vi "Generate write queue item.vi"(8 "error in (no error)":errorcluster, 10 "Request ID":u64, 11 "Register JSON in":refnum<class "Register JSON.lvclass">) -> (0 "error out":errorcluster, 2 "Write queue item":T1, 3 "Register JSON out":refnum<class "Register JSON.lvclass">)   [LabVIEW 2020, in "wamplv.lvlib" / "Register JSON.lvclass"]
uses:
  Register JSON.lvclass
  Register JSON.lvclass/Register JSON.ctl
  TypeDefs/WAMP Message Codes.ctl
  wamplv.lvlib
  Utils/Utils.lvclass
  91faa4a0-8572-4326-99ac-79b83bae1e0d.vi
  TypeDefs/Transport type.ctl
  WAMP Client/Private/TypeDef/Write queue item.ctl
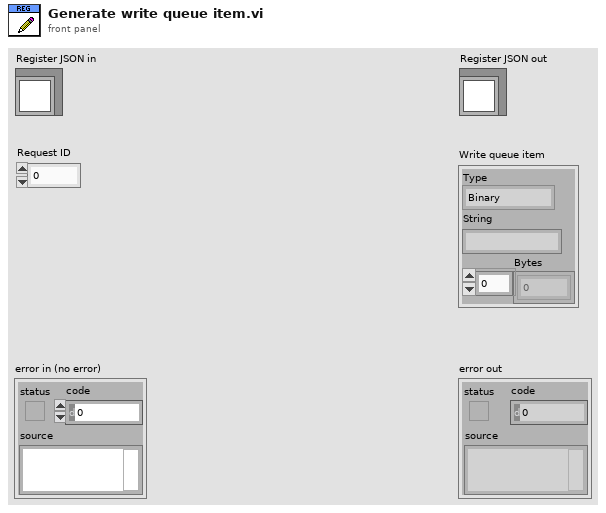
[diagram p1: front panel]
types:
  T1 = typedef "wamplv.lvlib/Write queue item.ctl" = cluster{"Type":T2, "String":string, "Bytes":u8[]}
  T2 = typedef "wamplv.lvlib/Transport type.ctl" = enum16{"Binary", "Text"}
  T3 = typedef "wamplv.lvlib/WAMP Message Codes.ctl" = enum8{"HELLO", "WELCOME", "CHALLENGE", "AUTHENTICATE", "ABORT", "GOODBYE", "ERROR", "PUBLISH", "PUBLISHED", "SUBSCRIBE", "SUBSCRIBED", "UNSUBSCRIBE", "UNSUBSCRIBED", "EVENT", "CALL", "RESULT", "REGISTER", "REGISTERED", "UNREGISTER", "UNREGISTERED", "INVOCATION", "YIELD"}
  T4 = typedef "wamplv.lvlib/REGISTER Request Data.ctl" = cluster{"Procedure URI":string, "Options":string, "REGISTER result notifier":refnum<notifier>}
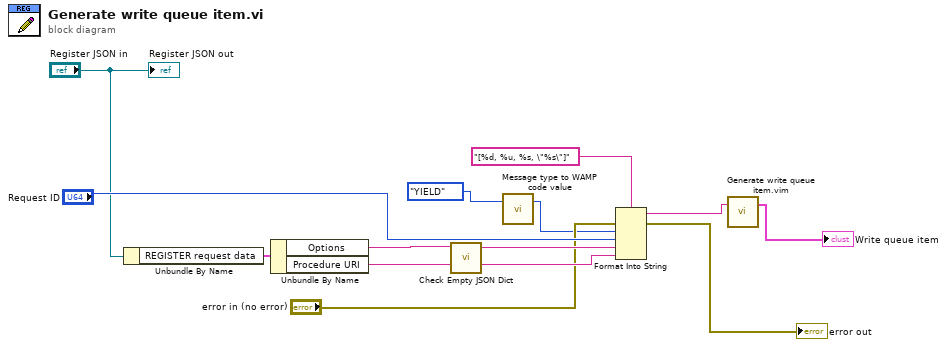
[diagram p0: block diagram]
diagram:
  n1 = Unbundle By Name("Register JSON in") -> ("REGISTER request data"=w6:T4)
  n2 = Unbundle By Name(w6) -> ("Options"=w12:string, "Procedure URI"=w11:string)
  n3 = call "Check Empty JSON Dict.vi"("JSON in"=w12) -> ("JSON out"=w13:string)  [unwired: 10 in]
  n4 = call "Message type to WAMP code value.vi"("Message Type"=WAMP_Message_Codes."YIELD" ("Message Codes")) -> ("WAMP Numeric value"=w1:u8)  [unwired: 2 in]
  n5 = Format Into String(format string="[%d, %u, %s, \"%s\"]" ("element"), error in="error in (no error)", w1, "Request ID", w13, w11) -> (resulting string=w4:string, error out=→"error out":errorcluster)  [unwired: 1 in]
  n6 = call "Generate write queue item.vim"("Input"=w4) -> ("Ouput"=→"Write queue item":T1)  [unwired: 2 in]
  "Register JSON out" <- "Register JSON in"
